vi "python_integration_vi.vi"() -> ()   [LabVIEW 2022 SP3]
panel:
  out "return value":i32
  in  "error in (no error)":errorcluster
  out "error out":errorcluster
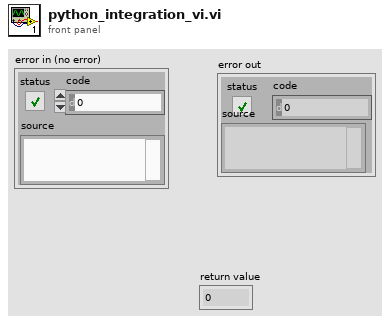
[diagram p1: front panel]
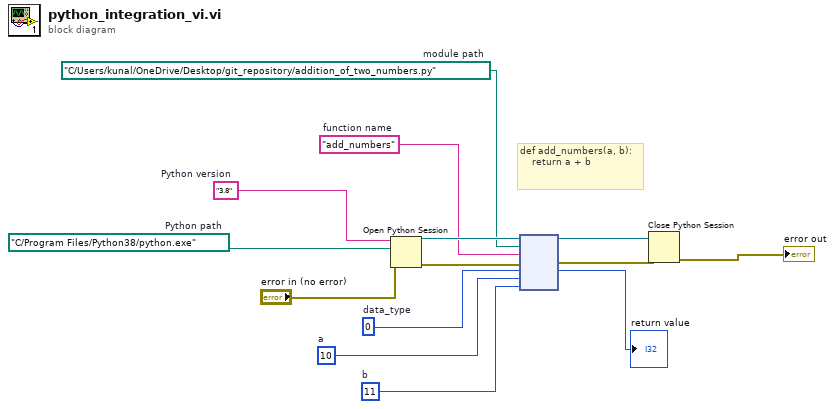
[diagram p0: block diagram]
diagram:
  w1 = 11  # b
  w2 = 10  # a
  w4 = 0  # data_type
  w5 = "add_numbers"  # function name
  w6 = path "C:/Users/kunal/OneDrive/Desktop/git_repository/addition_of_two_numbers.py"  # module path
  w8 = path "C:/Program Files/Python38/python.exe"  # Python path
  w9 = "3.8"  # Python version
  # "def add_numbers(a, b):\n    return a + b"
  n1 = Open Python Session(python version=w9, python path=w8, 3:"error in (no error)") -> (session out=w13:refnum<k35>, error out=w12:errorcluster)
  n2 = node(w13, w6, w5, w12, w4, w2, w1) -> (w14:refnum<k35>, w11:errorcluster, →"return value":i32)  [unwired: 2 in, 2 out]
  n3 = Close Python Session(session in=w14, error in=w11) -> (11:→"error out":errorcluster)
